vi "zero_set.vi"(10 "zero_set":bool, 11 "data_input":dbl[](array[numeric])) -> (3 "data_output":dbl[](array[numeric]))   [LabVIEW 2020]
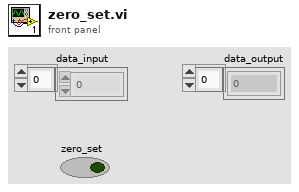
[diagram p1: front panel]
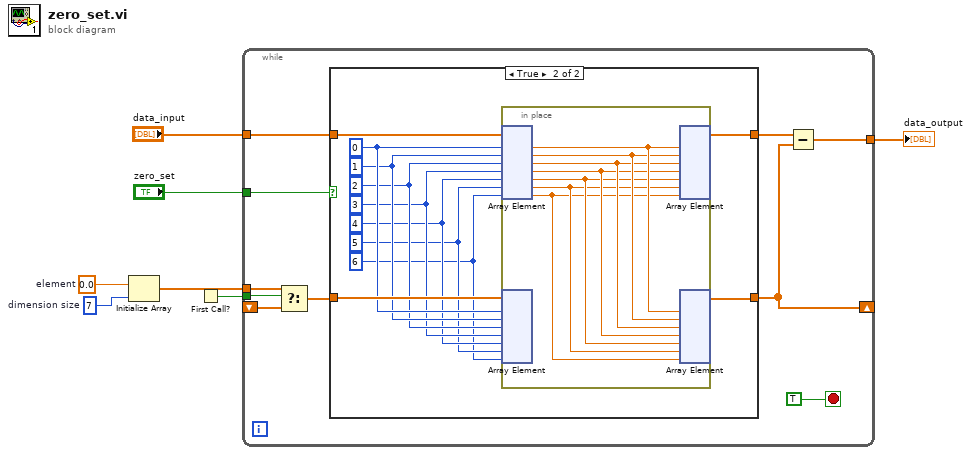
[diagram p0: block diagram]
diagram:
  w4 = 7  # dimension size
  w5 = 0.0  # element
  n1 = Initialize Array "Initialize Array"(w5, w4) -> (w2:dbl[])
  n2 = First Call?() -> (First Call?: T/F=w3:bool)
  n3 = while {
    tunnel: [w13] -> w7
    tunnel: "data_input" -> [w17]
    shift-right: [w14] -> _
    shift-left: _ -> [w11]
    tunnel: w3 -> [w12]
    tunnel: w2 -> [w10]
    tunnel: "zero_set" -> [w8]
    stop <- TRUE stop-if-true
    n4 = Select(t=w10, s=w12, f=w11) -> (s? t:f=w9:dbl[])
    n5 = case shown="True" w8 {
      tunnel: [w19 w30] -> w15
      tunnel: w17 -> [w19 w29]
      tunnel: w9 -> [w18 w28]
      tunnel: [w18 w27] -> w14
      frame False {
      }
      frame True {
        w20 = 6
        w21 = 5
        w22 = 4
        w23 = 3
        w24 = 2
        w25 = 1
        w26 = 0
        n6 = in-place {
          n7 = in-place-array #1(w29, w26, w25, w24, w23, w22, w21, w20) -> (w37:dbl, w36:dbl, w35:dbl, w34:dbl, w33:dbl, w32:dbl, w31:dbl)
          n8 = in-place-array #2(w28, w26, w25, w24, w23, w22, w21, w20) -> ()  [unwired: 7 out]
          n9 = in-place-array #1(w37, w36, w35, w34, w33, w32, w31) -> (w30:dbl[])  [unwired: 7 out]
          n10 = in-place-array #2(w37, w36, w35, w34, w33, w32, w31) -> (w27:dbl[])  [unwired: 7 out]
        }
      }
    }
    n11 = Subtract(x=w15, y=w14) -> (x-y=w13:dbl[])
  }
  "data_output" <- w7
